vi "stoperaseCI1_img.vi"   [LabVIEW 2013]
types:
  T1 = cluster{" CI1":refnum<k21>, "E_CI1":errorcluster}
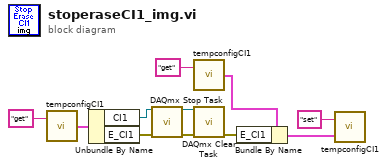
[diagram p0: block diagram]
diagram:
  n1 = call "tempconfigCI1.vi"("command"="get") -> ("Temp Config out"=w8:T1)  [unwired: 1 in]
  n2 = Unbundle By Name(w8) -> ("CI1"=w7:refnum<k21>, "E_CI1"=w6:errorcluster)
  n3 = call <vilib>:"DAQmx Stop Task.vi"("task/channels in"=w7, "error in"=w6) -> ("task out"=w10:refnum<k21>, "error out"=w11:errorcluster)  [unwired: 12 in]
  n4 = call "tempconfigCI1.vi"("command"="get") -> ("Temp Config out"=w3:T1)  [unwired: 1 in]
  n5 = call <vilib>:"DAQmx Clear Task.vi"("task in"=w10, "error in"=w11) -> ("error out"=w2:errorcluster)  [unwired: 13 in]
  n6 = Bundle By Name(cluster=w3, "E_CI1"=w2) -> (w1:T1)
  n7 = call "tempconfigCI1.vi"("Temp Config in"=w1, "command"="set") -> ()  [unwired: 1 out]
